vi "生成-报警记录缓存数据文件.vi"(8 "缓存绘图数据":cluster{"X":timestamp[], "Y":dbl[]}, 9 "限值":cluster{"限值1":dbl, "限值2":dbl}, 10 "探头信息":string, 11 "探头地址":i32) -> ()   [LabVIEW 2013]
uses:
  <vilib>/Utility/xml.llb/Write to XML File(string).vi
panel:
  out "结束时间2":string
  out "开始时间2":string
  out "结束时间1":string
  out "开始时间1":string
  out "结束2":timestamp
  out "开始2":timestamp
  out "结束1":timestamp
  out "开始1":timestamp
  out "最大值":string
  out "限值2":string
  out "限值1":string
  out "实时曲线":cluster{"X":timestamp[], "Y":dbl[]}[](graph)
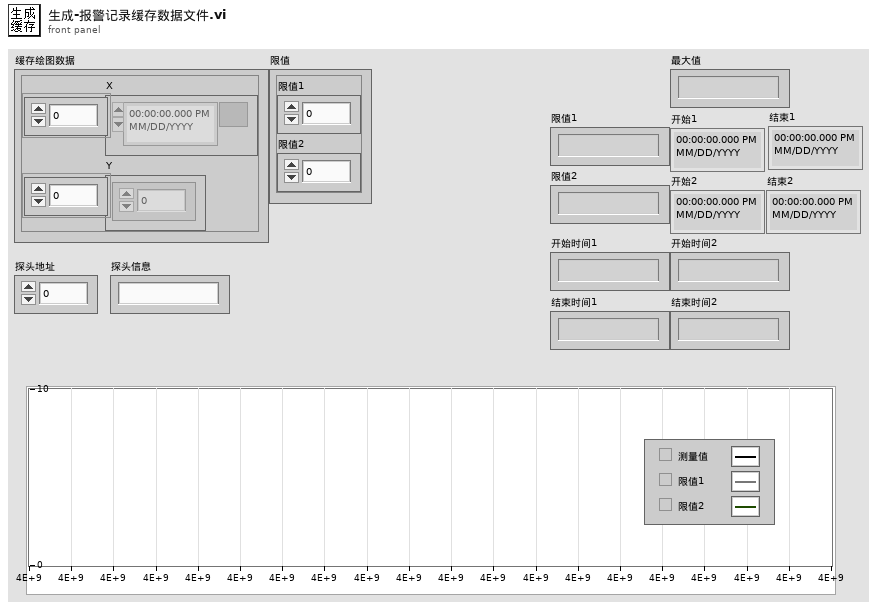
[diagram p1: front panel]
types:
  T1 = cluster{"限值":string, "报警时长":string, "最大值":string, "开始时间":string, "结束时间":string}
  T2 = cluster{"限值":string, "报警时长":string, "最大值":string, "开始时间":string, "结束时间":string}[]
  T3 = cluster{"实时曲线":cluster{"X":timestamp[], "Y":dbl[]}[], "书签-键-值":string[][]}
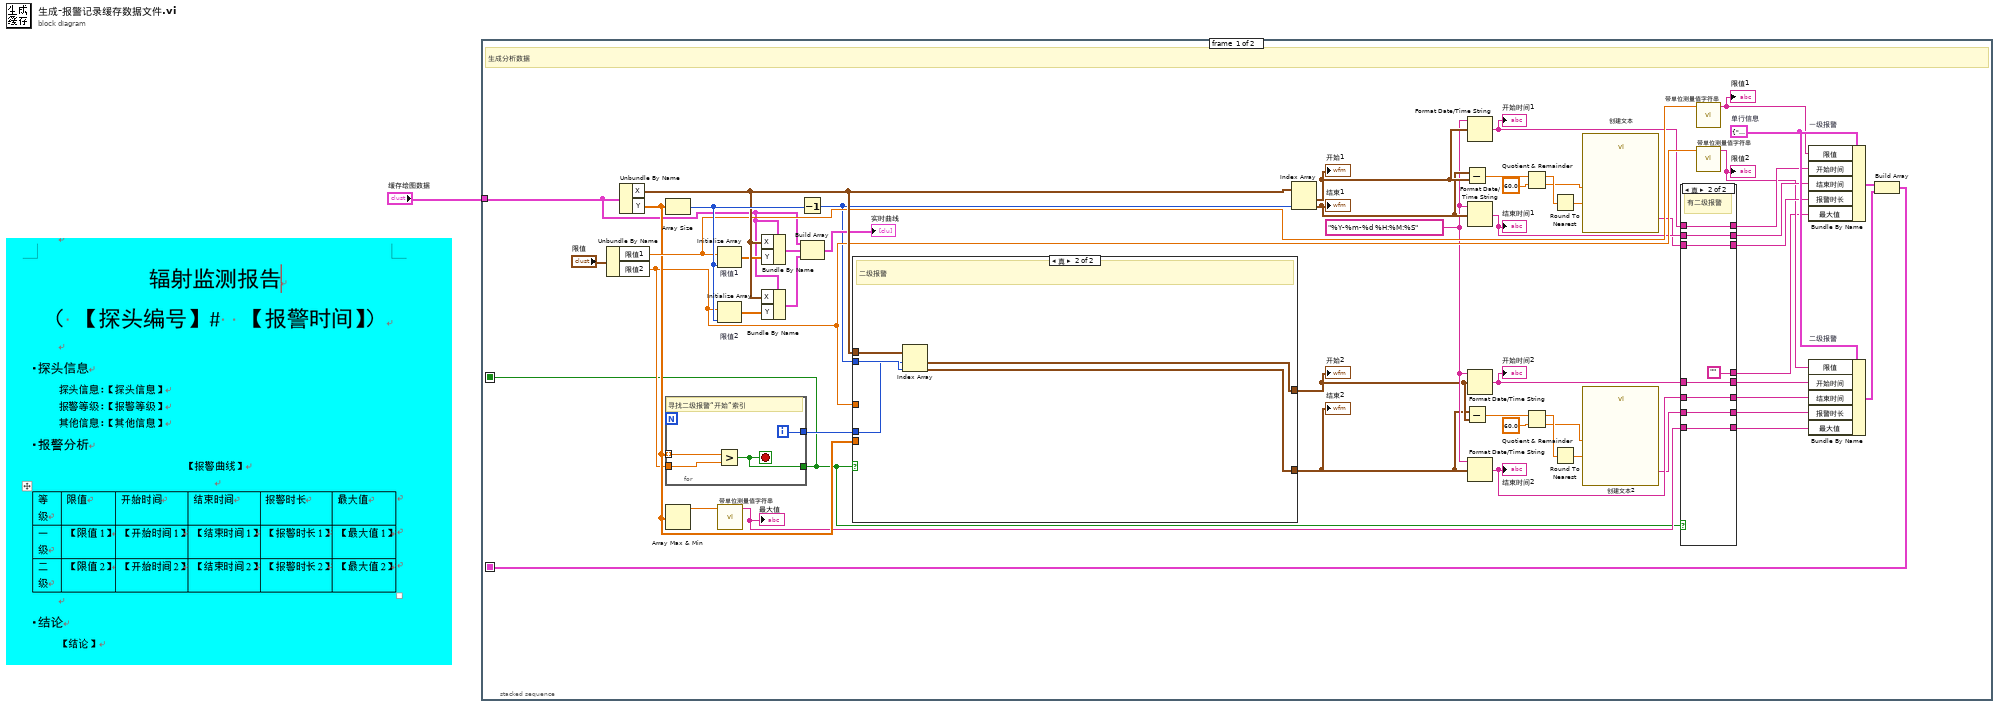
[diagram p0: block diagram]
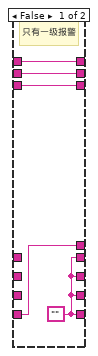
[diagram p2: hidden frame]
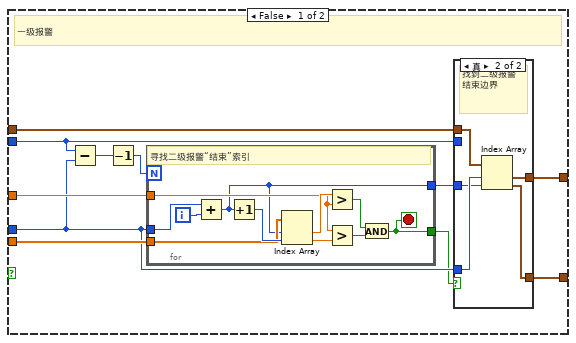
[diagram p3: hidden frame]
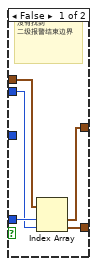
[diagram p4: hidden frame]
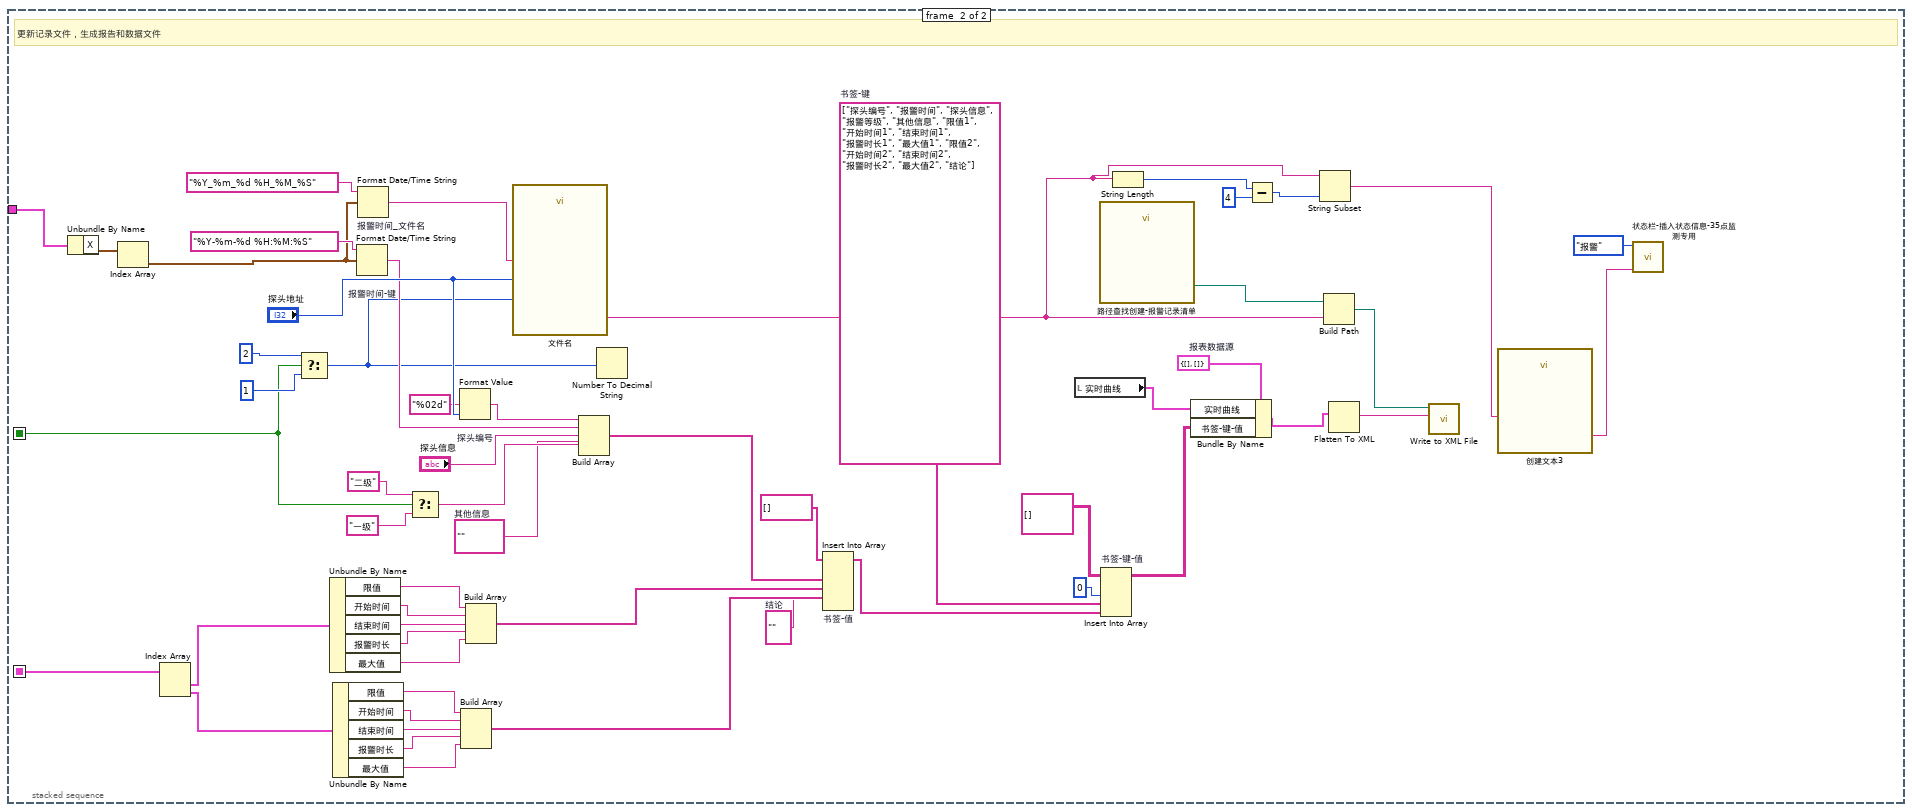
[diagram p5: hidden frame]
diagram:
  n1 = stacked-sequence {
    seq-local: [w4 _] -> [_ w148]
    seq-local: [w2 _] -> [_ w154]
    tunnel: "缓存绘图数据" -> [w3 w162]
    frame #0 {
      w34 = T1 {"限值"="", "报警时长"="", "最大值"="", "开始时间"="", "结束时间"=""}  # 单行信息
      w26 = "%Y-%m-%d %H:%M:%S" ("时间格式字符串(%c)")
      # "生成分析数据"
      n2 = Unbundle By Name("限值") -> ("限值1"=w45:dbl, "限值2"=w43:dbl)
      n3 = Unbundle By Name(w3) -> ("X"=w52:timestamp[], "Y"=w44:dbl[])
      n4 = Array Size(array=w44) -> (size(s)=w53:i32)
      n5 = for {
        tunnel: w44 -> [w107] mode=indexing
        tunnel: w43 -> [w106]
        tunnel: [w105] -> w42
        tunnel: [w104] -> w2
        i -> [w105]
        stop <- w104 stop-if-true
        # "寻找二级报警“开始”索引"
        n6 = Greater?(x=w107, y=w106) -> (0:w104:bool)
      }
      n7 = Array Max & Min(array=w44) -> (max value=w40:dbl)  [unwired: 3 out]
      n8 = Initialize Array "限值1"(w45, w53) -> (w51:dbl[])
      n9 = Initialize Array "限值2"(w43, w53) -> (w50:dbl[])
      n10 = call "带单位测量值字符串.vi"("测量值"=w40) -> ("结果"=w17:string)  [unwired: 10 in]
      "最大值" <- w17
      n11 = Bundle By Name(cluster=w3, "X"=w52, "Y"=w51) -> (w49:cluster{"X":timestamp[], "Y":dbl[]})
      n12 = Bundle By Name(cluster=w3, "X"=w52, "Y"=w50) -> (w48:cluster{"X":timestamp[], "Y":dbl[]})
      n13 = Decrement(x=w53) -> (x-1=w41:i32)
      n14 = Build Array(w3, w49, w48) -> (→"实时曲线":cluster{"X":timestamp[], "Y":dbl[]}[])
      n15 = case shown="真" w2 {
        tunnel: w52 -> [w73 w103]
        tunnel: w42 -> [w72 w99]
        tunnel: w44 -> [w77 _]
        tunnel: w43 -> [w76 _]
        tunnel: w41 -> [w69 w102]
        tunnel: [w68 w101] -> w25
        tunnel: [w67 w100] -> w24
        frame False {
          # "一级报警"
          n16 = Subtract(x=w69, y=w72) -> (x-y=w75:i32)
          n17 = Decrement(x=w75) -> (x-1=w74:i32)
          n18 = for {
            N: w74 -> [_]
            tunnel: w72 -> [w97]
            tunnel: w77 -> [w95]
            tunnel: w76 -> [w93]
            tunnel: [w89] -> w71
            tunnel: [w88] -> w70
            i -> [w98]
            stop <- w88 stop-if-true
            # "寻找二级报警“结束”索引"
            n19 = Add(x=w97, y=w98) -> (x+y=w89:i32)
            n20 = Increment(x=w89) -> (x+1=w96:i32)
            n21 = Index Array(array=w95, index #1=w89, index #2=w96) -> (element #1=w94:dbl, element #2=w92:dbl)
            n22 = Greater?(x=w94, y=w93) -> (0:w91:bool)
            n23 = Greater?(x=w93, y=w92) -> (0:w90:bool)
            n24 = And(x=w91, y=w90) -> (x .and. y?=w88:bool)
          }
          n25 = case shown="真" w70 {
            tunnel: w73 -> [w82 w87]
            tunnel: w72 -> [w81 w86]
            tunnel: w71 -> [_ w85]
            tunnel: [w80 w84] -> w68
            tunnel: [w78 w83] -> w67
            tunnel: w69 -> [w79 _]
            frame False {
              # "没有找到\n二级报警结束边界"
              n26 = Index Array(array=w82, index #1=w81, index #2=w79) -> (element #1=w80:timestamp, element #2=w78:timestamp)
            }
            frame True {
              # "找到二级报警\n结束边界"
              n27 = Index Array(array=w87, index #1=w86, index #2=w85) -> (element #1=w84:timestamp, element #2=w83:timestamp)
            }
          }
        }
        frame True {
          # "二级报警"
          n28 = Index Array(array=w103, index #1=w99, index #2=w102) -> (element #1=w101:timestamp, element #2=w100:timestamp)
        }
      }
      "开始2" <- w25
      "结束2" <- w24
      n29 = Index Array(array=w52, index #2=w41) -> (element #1=w28:timestamp, element #2=w27:timestamp)  [unwired: 1 in]
      "开始1" <- w28
      "结束1" <- w27
      n30 = Subtract(x=w27, y=w28) -> (x-y=w39:dbl)
      n31 = Subtract(x=w24, y=w25) -> (x-y=w31:dbl)
      n32 = Format Date/Time String(time format string (%c)=w26, seconds (now)=w28) -> (date/time string=w22:string)  [unwired: 1 in]
      "开始时间1" <- w22
      n33 = Format Date/Time String(time format string (%c)=w26, seconds (now)=w27) -> (date/time string=w20:string)  [unwired: 1 in]
      "结束时间1" <- w20
      n34 = Format Date/Time String(time format string (%c)=w26, seconds (now)=w25) -> (date/time string=w7:string)  [unwired: 1 in]
      "开始时间2" <- w7
      n35 = Format Date/Time String(time format string (%c)=w26, seconds (now)=w24) -> (date/time string=w6:string)  [unwired: 1 in]
      "结束时间2" <- w6
      n36 = Quotient & Remainder(x=w39, y=60.0) -> (x-y*floor(x/y)=w37:dbl, floor(x/y)=w35:dbl)
      n37 = Quotient & Remainder(x=w31, y=60.0) -> (x-y*floor(x/y)=w33:dbl, floor(x/y)=w29:dbl)
      n38 = Round To Nearest(number=w37) -> (nearest integer value=w36:dbl)
      n39 = Round To Nearest(number=w33) -> (nearest integer value=w30:dbl)
      n40 = call "创建文本"("分"=w35, "秒"=w36) -> ("Result"=w18:string)  [unwired: 12 in, 1 out]
      n41 = call "创建文本2"("分"=w29, "秒"=w30) -> ("Result"=w5:string)  [unwired: 12 in, 1 out]
      n42 = case shown="真" w2 {
        tunnel: [w58 w65] -> w23
        tunnel: w22 -> [w58 w65]
        tunnel: [w57 w64] -> w21
        tunnel: w20 -> [w57 w64]
        tunnel: [w56 w63] -> w19
        tunnel: w18 -> [w56 w63]
        tunnel: w17 -> [w55 w59]
        tunnel: [w55 ""] -> w14
        tunnel: [w54 w62] -> w11
        tunnel: [w54 w61] -> w10
        tunnel: [w54 w60] -> w9
        tunnel: [w54 w59] -> w8
        tunnel: w7 -> [_ w62]
        tunnel: w6 -> [_ w61]
        tunnel: w5 -> [_ w60]
        frame False {
          w54 = ""
          # "只有一级报警"
        }
        frame True {
          # "有二级报警"
        }
      }
      n43 = call "带单位测量值字符串.vi"("测量值"=w45) -> ("结果"=w16:string)  [unwired: 10 in]
      "限值1" <- w16
      n44 = call "带单位测量值字符串.vi"("测量值"=w43) -> ("结果"=w15:string)  [unwired: 10 in]
      "限值2" <- w15
      n45 = Bundle By Name "一级报警"(cluster=w34, "限值"=w16, "开始时间"=w23, "结束时间"=w21, "报警时长"=w19, "最大值"=w14) -> (w13:T1)
      n46 = Bundle By Name "二级报警"(cluster=w34, "限值"=w15, "开始时间"=w11, "结束时间"=w10, "报警时长"=w9, "最大值"=w8) -> (w12:T1)
      n47 = Build Array(w13, w12) -> (w4:T2)
    }
    frame #1 {
      w126 = T3 {"实时曲线"=[], "书签-键-值"=[]}  # 报表数据源
      w128 = string[] ["探头编号", "报警时间", "探头信息", "报警等级", "其他信息", "限值1", "开始时间1", "结束时间1", "报警时长1", "最大值1", "限值2", "开始时间2", "结束时间2", "报警时长2", "最大值2", "结论"]  # 书签-键
      w131 = ""  # 结论
      w149 = ""  # 其他信息
      # "更新记录文件，生成报告和数据文件"
      n48 = Unbundle By Name(w162) -> ("X"=w161:timestamp[])
      n49 = Index Array(array=w161) -> (element=w116:timestamp)  [unwired: 1 in]
      n50 = Index Array(array=w148) -> (element #1=w147:T1, element #2=w146:T1)  [unwired: 2 in]
      n51 = Select(t=2, s=w154, f=1) -> (s? t:f=w118:i32)
      n52 = Unbundle By Name(w147) -> ("限值"=w145:string, "开始时间"=w144:string, "结束时间"=w143:string, "报警时长"=w142:string, "最大值"=w141:string)
      n53 = Unbundle By Name(w146) -> ("限值"=w140:string, "开始时间"=w139:string, "结束时间"=w138:string, "报警时长"=w137:string, "最大值"=w136:string)
      n54 = Format Date/Time String "报警时间-键"(time format string (%c)="%Y-%m-%d %H:%M:%S" ("时间格式字符串(%c)"), seconds (now)=w116) -> (date/time string=w120:string)  [unwired: 1 in]
      n55 = Format Date/Time String "报警时间_文件名"(time format string (%c)="%Y_%m_%d %H_%M_%S" ("时间格式字符串(%c)"), seconds (now)=w116) -> (date/time string=w115:string)  [unwired: 1 in]
      n56 = Select(t="二级" ("格式字符串"), s=w154, f="一级" ("格式字符串")) -> (s? t:f=w150:string)
      n57 = Format Value "探头编号"(format string="%02d" ("格式字符串"), value (0)="探头地址") -> (output string=w119:string)  [unwired: 1 in]
      n58 = Build Array(w140, w139, w138, w137, w136) -> (w132:string[])
      n59 = Build Array(w145, w144, w143, w142, w141) -> (w133:string[])
      n60 = call "文件名"("时间"=w115, "探头地址XX"="探头地址", "报警等级"=w118) -> ("Result"=w109:string)  [unwired: 11 in, 1 out]
      n61 = Build Array(w119, w120, "探头信息", w150, w149) -> (w135:string[])
      n62 = Number To Decimal String(number=w118) -> ()  [unwired: 1 in, 1 out]
      n63 = Insert Into Array "书签-值"(array=string[] [] ("数组"), new element #1=w135, new element #2=w133, new element #3=w132, new element #4=w131) -> (w127:string[])  [unwired: 1 in]
      n64 = local read "实时曲线"() -> (w125:cluster{"X":timestamp[], "Y":dbl[]}[])
      n65 = call "路径查找创建-报警记录清单.vi"() -> ("缓存数据文件夹"=w159:path)  [unwired: 6 in, 5 out]
      n66 = Insert Into Array "书签-键-值"(array=string[][] [] ("数组"), index (col)=0 ("禁用的索引 (列)"), new element #1=w128, new element #2=w127) -> (w124:string[][])  [unwired: 1 in]
      n67 = String Length(string=w109) -> (length=w112:i32)
      n68 = Bundle By Name(cluster=w126, "实时曲线"=w125, "书签-键-值"=w124) -> (w123:T3)
      n69 = Subtract(x=w112, y=4) -> (x-y=w110:i32)
      n70 = String Subset(string=w109, length (rest)=w110) -> (substring=w108:string)  [unwired: 1 in]
      n71 = Build Path(base path=w159, name or relative path=w109) -> (appended path=w122:path)
      n72 = Flatten To XML(anything=w123) -> (xml string=w121:string)
      n73 = call-poly <vilib>:"Write to XML File.vi"("XML Input"=w121, "XML File Path"=w122) -> ()  [unwired: 7 in, 3 out]
      n74 = call "创建文本3"("文件名"=w108) -> ("Result"=w113:string)  [unwired: 13 in, 1 out]
      n75 = call "状态栏-插入状态信息-35点监测专用.vi"("消息内容"=w113, "状态类型"=enum16{"全部", "报警", "通信", "设置"}."报警") -> ()  [unwired: 10 in]
    }
  }
